vi "Test_Log.vi"(8 "error in":errorcluster, 10 "directory":path, 11 "minimum log level":T4=enum."Info") -> (0 "error out":errorcluster, 3 "failure info":T1 {"Log Record"."timestamp" format="%<%x %.3X>T"})   [LabVIEW 2018]
uses:
  api/Log Levels.ctl
  api/Failure Information.ctl
  api/Log Record.ctl
  api/logger_class/Internal Log Levels.ctl
  api/configuration/formatters/format_string_formatter/Format String.lvclass
  C:/Users/Colin/Documents/software_projects/labview/glog/src/api/extension/formatter_interface/Formatter.lvclass
  api/configuration/handlers/file_handler/File Handler.lvclass
  C:/Users/Colin/Documents/software_projects/labview/glog/src/api/extension/formatting_handler_interface/Formatting Handler.lvclass
  api/logger_class/Log (Parts).vi
  api/logger_class/Logger.lvclass
  api/GLog.lvlib
panel:
  # "Connector Pane"
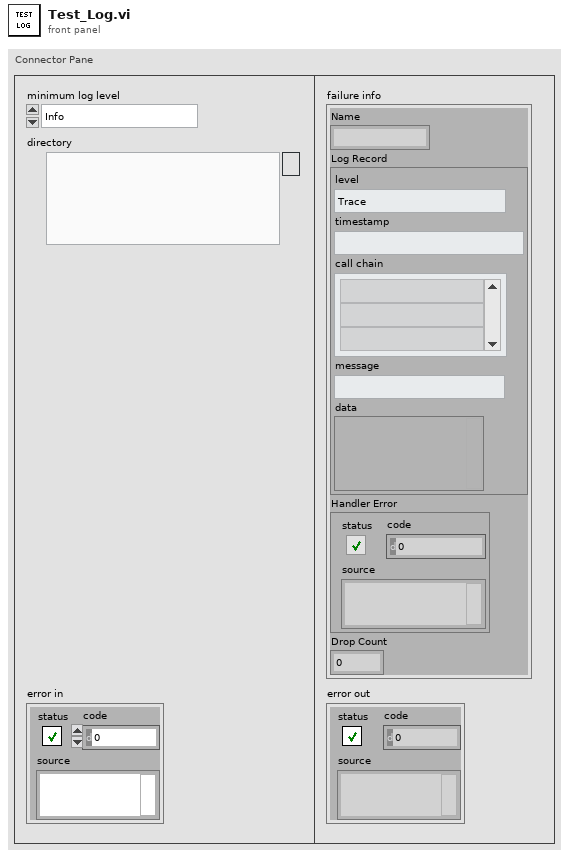
[diagram p1: front panel]
types:
  T1 = typedef "GLog.lvlib/Failure Information.ctl" = cluster{"Name":string, "Log Record":T2, "Handler Error":errorcluster, "Drop Count":u32}
  T2 = typedef "GLog.lvlib/Log Record.ctl" = cluster{"level":T3, "timestamp":timestamp, "call chain":string[], "message":string, "data":variant}
  T3 = typedef "GLog.lvlib/Internal Log Levels.ctl" = enum16{"Trace", "Debug", "Info", "Warning", "Error", "Critical", "Internal"}
  T4 = typedef "GLog.lvlib/Log Levels.ctl" = enum16{"Trace", "Debug", "Info", "Warning", "Error", "Critical"}
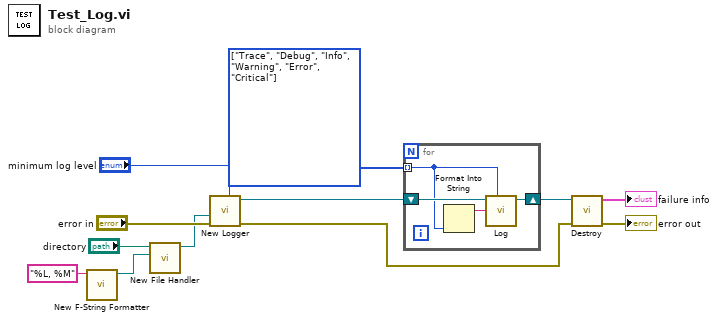
[diagram p0: block diagram]
diagram:
  w12 = T4[] [enum."Trace", enum."Debug", enum."Info", enum."Warning", enum."Error", enum."Critical"] items=["Trace", "Debug", "Info", "Warning", "Error", "Critical"] ("Array")
  n1 = call "New F-String Formatter.vi"("format string (\"%T | %L | %M\")"="%L, %M" ("format string (\"%T | %L | %M\")")) -> ("new f-string formatter"=w3:refnum<class "Format String.lvclass">)  [unwired: 10 in]
  n2 = call "New File Handler.vi"("formatter (JSON)"=w3, "log directory (<app dir>/logs)"="directory") -> ("file handler"=w4:refnum<class "File Handler.lvclass">)  [unwired: 9 in]
  n3 = call "New Logger.vi"("minimum log level (Info)"="minimum log level", "error in (no error)"="error in", "log handler (file handler)"=w4) -> ("error out"=w7:errorcluster, "logger"=w11:refnum<class "Logger.lvclass">)  [unwired: 7 in]
  n4 = for {
    tunnel: w12 -> [w13] mode=indexing
    shift-right: [w15] -> w10
    shift-left: w11 -> [w16]
    n5 = Format Into String(w13) -> (resulting string=w14:string)  [unwired: 3 in, 1 out]
    n6 = call-poly "Log.vi"("log level"=w13, "message"=w14, "logger in"=w16) -> ("logger out"=w15:refnum<class "Logger.lvclass">)  [unwired: 8 in]
  }
  n7 = call "Destroy.vi"("error in (no error)"=w7, "logger in"=w10) -> ("error out"=→"error out":errorcluster, "failure info"=→"failure info":T1)  [unwired: 8 in]
